vi "After Launch Init Core.vi"(8 "error in (no error)":errorcluster, 11 "CS++GoBangClient in":refnum<class "CS++GoBangClient.lvclass">) -> (0 "error out":errorcluster, 3 "CS++GoBangClient out":refnum<class "CS++GoBangClient.lvclass">)   [LabVIEW 2014, in "GoBang.lvlib" / "CS++GoBangClient.lvclass"]
doc: "Use <b>Pre Launch init.vi</b> method only for sanity checks that are supposed to prevent the actor from launching if they fail. Use <B>this</B> method instead to initialize unique resources that must be released during the <b>Stop Core.vi</b> method. A corresponding high priority message will become dispatched before the <B>Actor Framework.lvlib:Actor.lvclass.Actor Core.vi</b> is called.\n\n<b>Derived classed should call the parent methode first</b> and their own initialization code after.\n\nRefer also to the ongoing discussion at https://decibel.ni.com/content/message/57394#57394."
uses:
  CS++GoBangClient.lvclass
  CSPP_Core/Classes/CS++ProcessVariables/PVConnection/PVConnection.lvclass
  CSPP_Core/Actors/CS++BaseActor/CS++BaseActor.lvclass
  CSPP_Core/Classes/CS++ProcessVariables/ProcessVariable/PV.lvclass
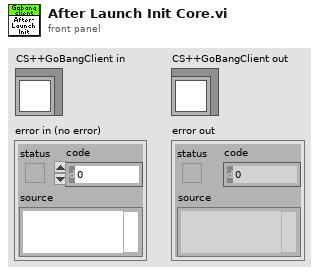
[diagram p1: front panel]
types:
  T1 = cluster{"Write Access":enum8{"Allowed", "Required", "None"}, "Read Access":enum8{"Allowed", "Required", "None"}}
  T2 = cluster{"JoinGame":refnum<class "PVConnection.lvclass">, "UpdateBoard":refnum<class "PVConnection.lvclass">}
  T3 = cluster{"[0]":refnum<class "PVConnection.lvclass">, "[1]":refnum<class "PVConnection.lvclass">}
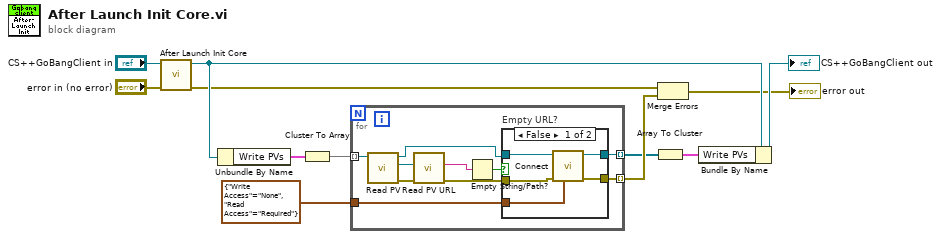
[diagram p0: block diagram]
diagram:
  n1 = call-parent "After Launch Init Core.vi"("error in (no error)"="error in (no error)", "CS++BaseActor in"="CS++GoBangClient in") -> ("error out"=w1:errorcluster, "CS++BaseActor out"=w4:refnum<class "CS++GoBangClient.lvclass">)  [unwired: 8 in]
  n2 = Unbundle By Name(w4) -> ("Write PVs"=w6:T2)
  n3 = Cluster To Array(cluster=w6) -> (array=w8:refnum<class "PVConnection.lvclass">[])
  n4 = for {
    tunnel: w8 -> [w18] mode=indexing
    tunnel: T1 {"Write Access"=enum."None", "Read Access"=enum."Required"} ("Access") -> [w22]
    tunnel: [w21] -> w9 mode=indexing
    tunnel: [w19] -> w10 mode=indexing
    n5 = call "Read PV.vi"("PVConnection in"=w18) -> ("error out"=w16:errorcluster, "PV"=w17:refnum<class "PV.lvclass">, "PVConnection out"=w13:refnum<class "PVConnection.lvclass">)  [unwired: 8 in]
    n6 = call "Read PV URL.vi"("error in (no error)"=w16, "PV in"=w17) -> ("error out"=w15:errorcluster, "PV URL"=w14:string)  [unwired: 7 in, 1 out]
    n7 = Empty String/Path?(string/path=w14) -> (empty?=w20:bool)
    n8 = case "Empty URL?" shown="False" w20 {
      tunnel: w13 -> [w27 w28]
      tunnel: w22 -> [w25 _]
      tunnel: [w26 w28] -> w21
      tunnel: [w24 _] -> w19
      tunnel: w15 -> [w23 _]
      frame False {
        n9 = call "Connect.vi"("Access (R/W allowed)"=w25, "error in (no error)"=w23, "PVConnection in"=w27) -> ("error out"=w24:errorcluster, "PVConnection out"=w26:refnum<class "PVConnection.lvclass">)  [unwired: 7 in]
      }
      frame True {
      }
    }
  }
  n10 = Array To Cluster(array=w9) -> (cluster=w7:T3)
  n11 = Merge Errors(w1, w10) -> (→"error out":errorcluster)
  n12 = Bundle By Name(cluster=w4, "Write PVs"=w7) -> (→"CS++GoBangClient out":refnum<class "CS++GoBangClient.lvclass">)
